vi "5p1_HW_Task1_UCweesesr.vi"() -> ()   [LabVIEW 2016]
panel:
  out "Force":string
  in  "Distance (in meters)":dbl
  in  "Coulumbs 2 (in C)":dbl
  in  "Coulumbs 1 (in C)":dbl
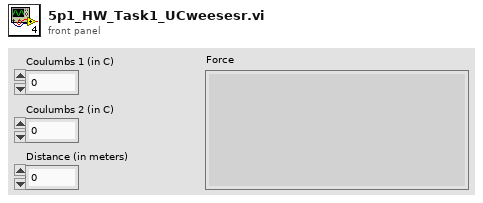
[diagram p1: front panel]
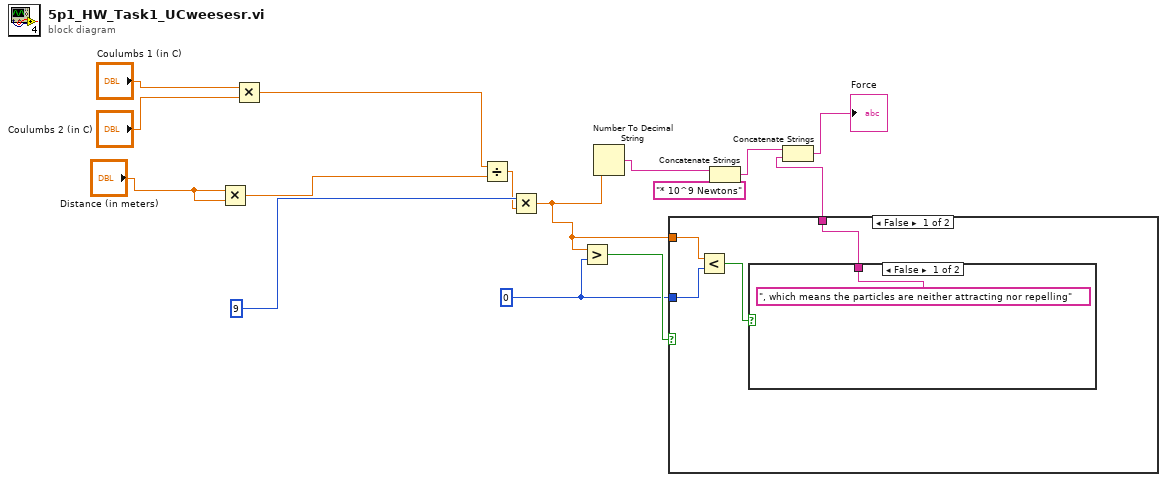
[diagram p0: block diagram]
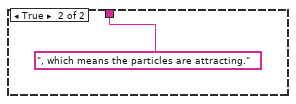
[diagram p2: hidden frame]
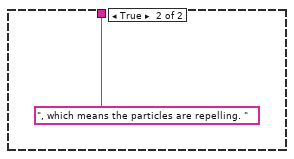
[diagram p3: hidden frame]
diagram:
  w4 = 0
  n1 = Multiply(x="Distance (in meters)", y="Distance (in meters)") -> (x*y=w12:dbl)
  n2 = Multiply(x="Coulumbs 1 (in C)", y="Coulumbs 2 (in C)") -> (x*y=w11:dbl)
  n3 = Divide(x=w11, y=w12) -> (x/y=w9:dbl)
  n4 = Multiply(x=9, y=w9) -> (x*y=w5:dbl)
  n5 = Greater?(x=w5, y=w4) -> (0:w7:bool)
  n6 = Number To Decimal String(number=w5) -> (decimal integer string=w3:string)  [unwired: 1 in]
  n7 = case shown="False" w7 {
    tunnel: [w16 ", which means the particles are repelling. "] -> w6
    tunnel: w5 -> [w19 _]
    tunnel: w4 -> [w18 _]
    frame False {
      n8 = Less?(x=w19, y=w18) -> (x < y?=w17:bool)
      n9 = case shown="False" w17 {
        tunnel: [", which means the particles are neither attracting nor repelling" ", which means the particles are attracting."] -> w16
        frame False {
        }
        frame True {
        }
      }
    }
    frame True {
    }
  }
  n10 = Concatenate Strings(w3, "* 10^9 Newtons") -> (w2:string)
  n11 = Concatenate Strings(w2, w6) -> (→"Force":string)
